vi "Image Difference Main Page.vi"(8 "error in (no error)":errorcluster, 11 "Node Ptr":T3 format="%.0x") -> (0 "error out":errorcluster)   [LabVIEW 2012, in "Image Difference Custom Device.lvlib"]
uses:
  Image Difference Custom Device.lvlib
  <vilib>/NI Veristand/Custom Device API/Custom Device Item Ref.ctl
  <vilib>/userdefined/High Color/IMAQdx.ctl
  TypeDefs/Image Difference State Variables.ctl
  <vilib>/vision/Image Controls.llb/IMAQ Image.ctl
  <vilib>/NI/AMC/Read Next Message.vi
  <vilib>/NI/AMC/Send Local Message.vi
  <vilib>/NI/AMC/Send Local Messages.vi
  <vilib>/NI/AMC/Read Termination Message.vi
  <vilib>/NI/AMC/Create Single Message.vi
  <vilib>/NI/AMC/Update Message Routing Info.vi
  <vilib>/NI/AMC/Create Multiple Messages.vi
  <vilib>/NI/AMC/Create Message Queue.vi
  <vilib>/NI/AMC/Globals.vi
  <vilib>/NI/AMC/Send Message.vi
  Image Difference Global.vi
  <vilib>/NI Veristand/Custom Device API/Set Item Property (String).vi
  <vilib>/NI Veristand/Custom Device API/Set Item Property (Variant).vi
  <vilib>/NI Veristand/Custom Device API/Get Item Property (Variant).vi
  <vilib>/NI Veristand/Custom Device API/Get Item Property (String).vi
  <vilib>/NI/AMC/Destroy Message Queue.vi
  <vilib>/NI Veristand/Custom Device API/Custom Device API.lvlib
  <vilib>/vision/driver/NI_Vision_Acquisition_Software.lvlib
panel:
  in  "Snap Camera":bool
  in  "Camera Session":T1 caption="Session Out"
  out "Camera Image":T2(plugin-control)
  in  "Reset ROI":bool
  in  "Commit ROI":bool
  in  "LoadImage":bool
  in  "Header":cluster{"Section Name":string}={"Section Name"="Custom Device Item Settings"}
  in  "Name":string
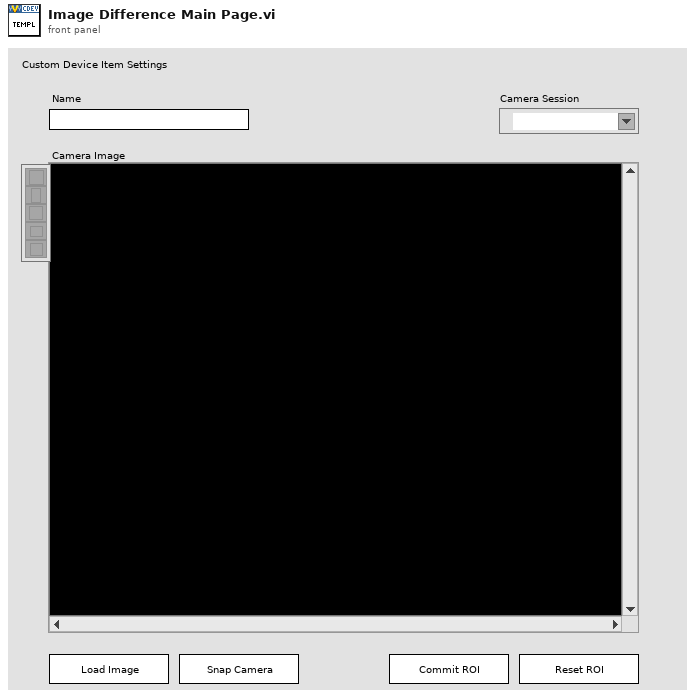
[diagram p1: front panel]
types:
  T1 = typedef "IMAQdx.ctl" = refnum<k21>
  T2 = typedef "IMAQ Image.ctl" = refnum<image>
  T3 = typedef "Custom Device API.lvlib/Custom Device Item Ref.ctl" = u64
  T4 = typedef "Image Difference Custom Device.lvlib/Image Difference State Variables.ctl" = cluster{"NIVS Event":refnum<event-registration>, "Image ROI":cluster{"Global Rectangle":i32[], "Contours":cluster{"Contour Type":u32, "ROI Type":u32, "Points":i32[]}[]}, "Camera Image":T2, "Mouse Depressed?":bool, "Camera Path":string}
  T5 = typedef "AMC.lvlib/Message Queue.ctl" = refnum<queue>
  T6 = typedef "Custom Device API.lvlib/Custom Device Commands.ctl" = enum16{"Default", "Item renamed", "Shutdown", "Dynamic button pressed"}
  T7 = typedef "Custom Device API.lvlib/Custom Device Item Info.ctl" = cluster{"Name":string, "Is Channel":bool, "GUID":string, "Is Waveform":bool}
  T8 = cluster{"Global Rectangle":i32[], "Contours":cluster{"Contour Type":u32, "ROI Type":u32, "Points":i32[]}[]}
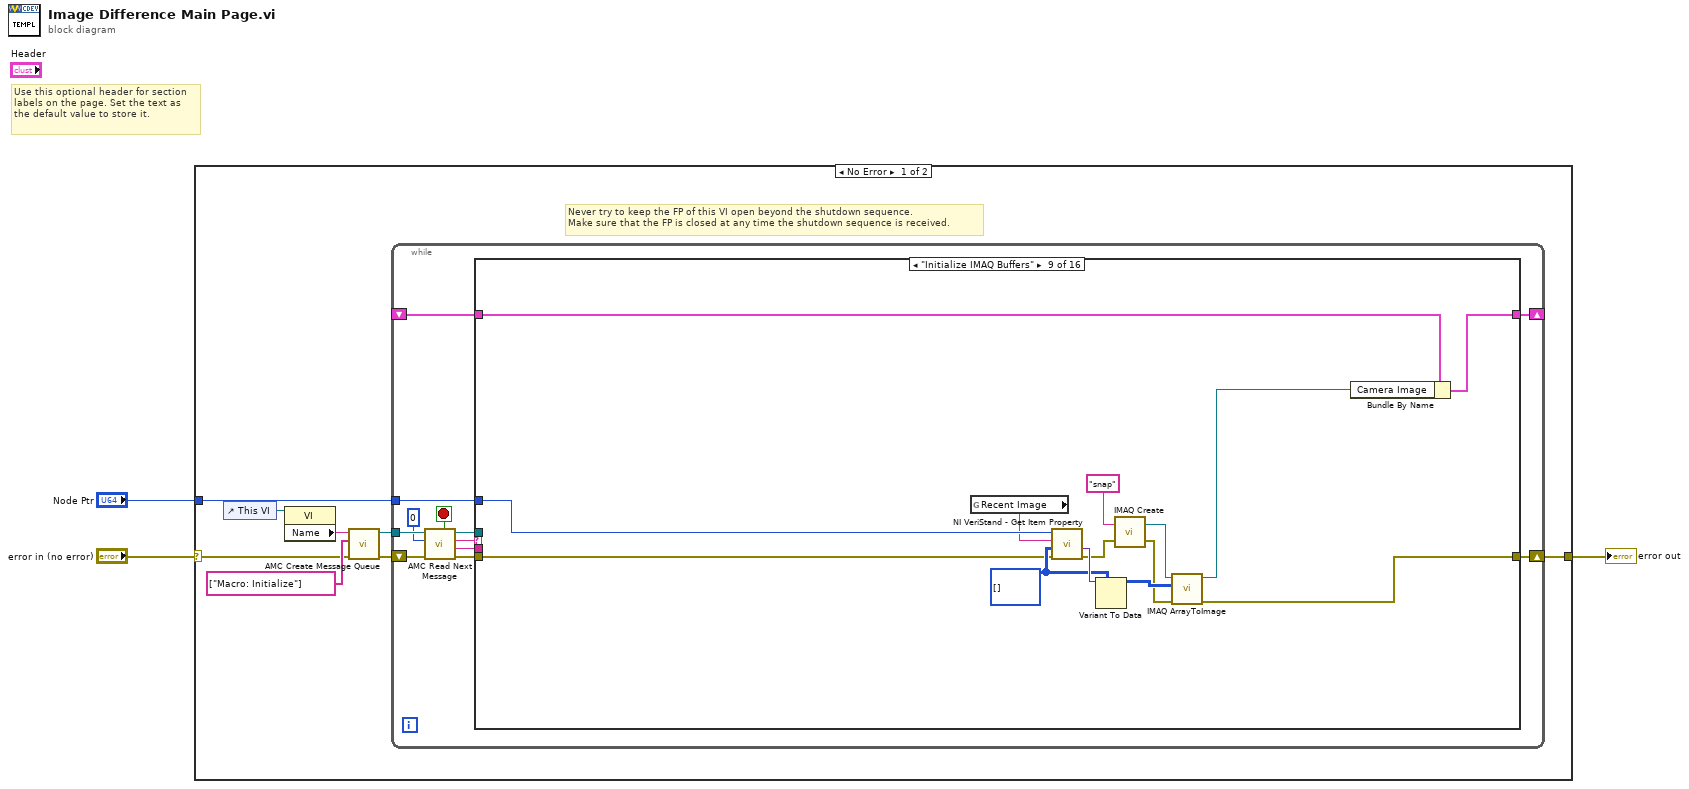
[diagram p0: block diagram]
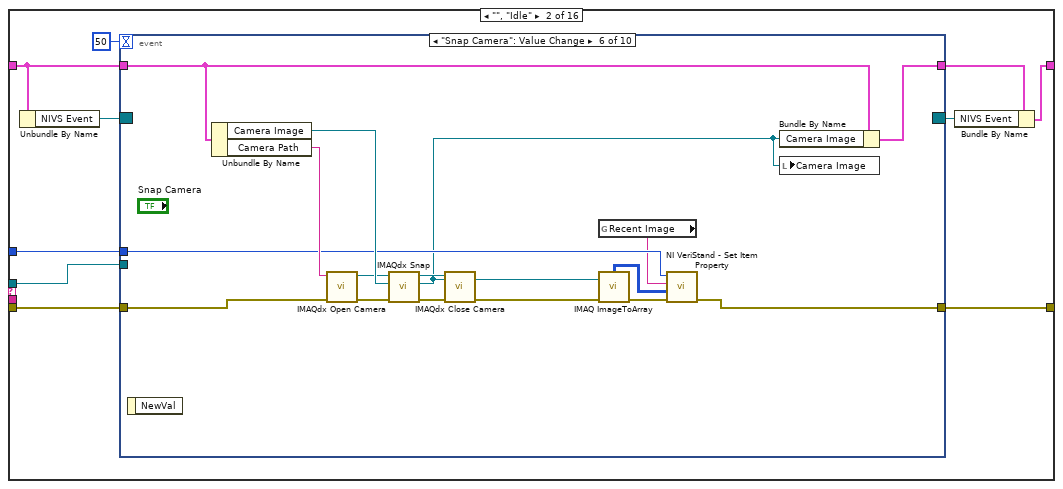
[diagram p3: hidden frame]
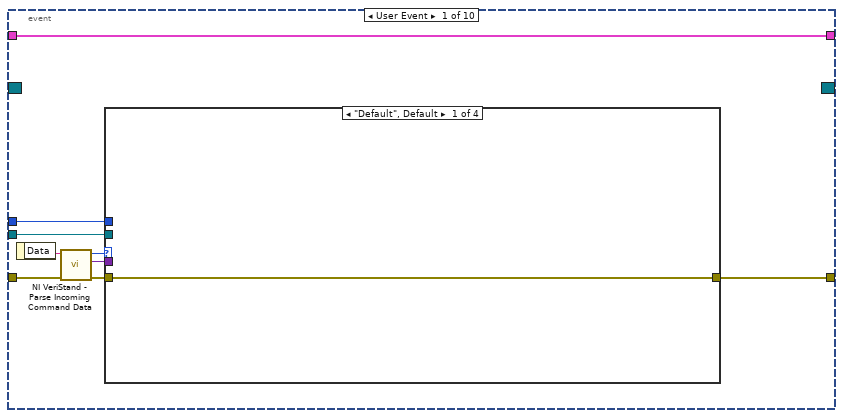
[diagram p4: hidden frame]
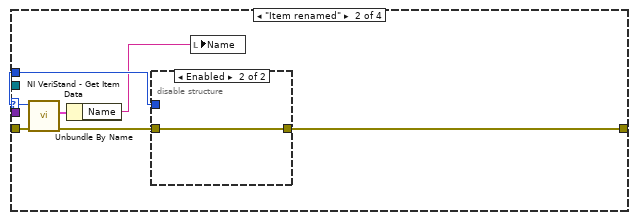
[diagram p5: hidden frame]
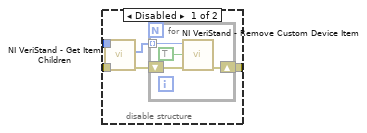
[diagram p6: hidden frame]
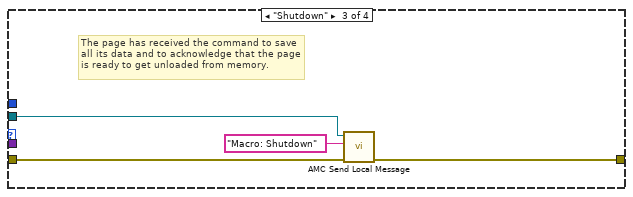
[diagram p7: hidden frame]
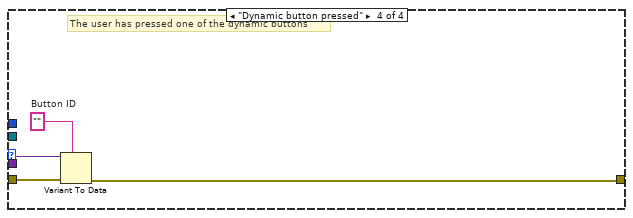
[diagram p8: hidden frame]
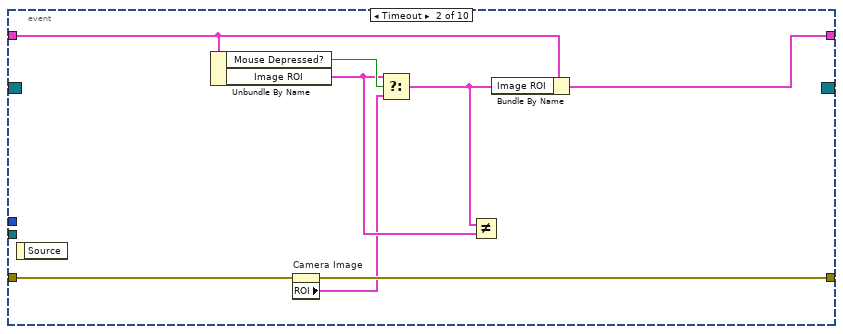
[diagram p9: hidden frame]
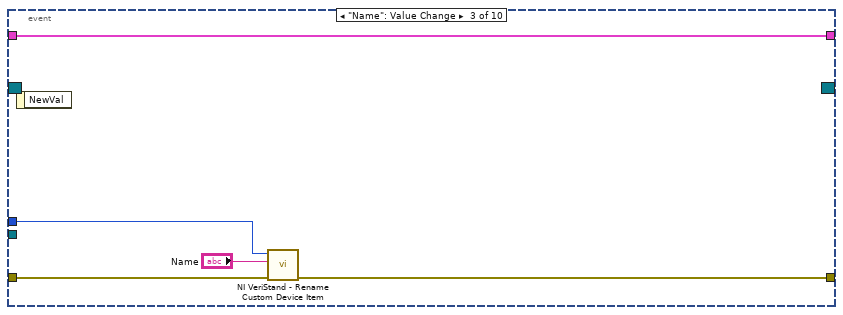
[diagram p10: hidden frame]
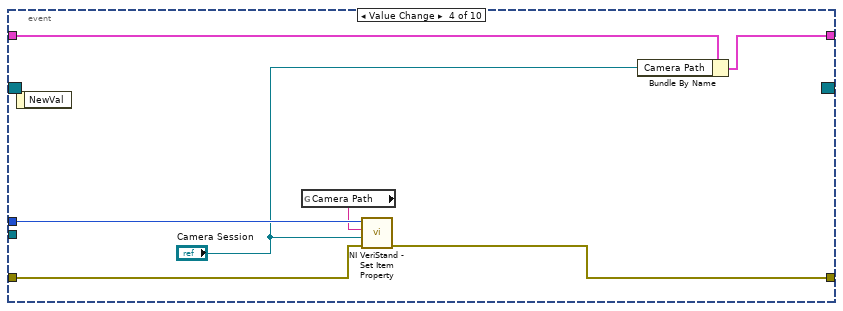
[diagram p11: hidden frame]
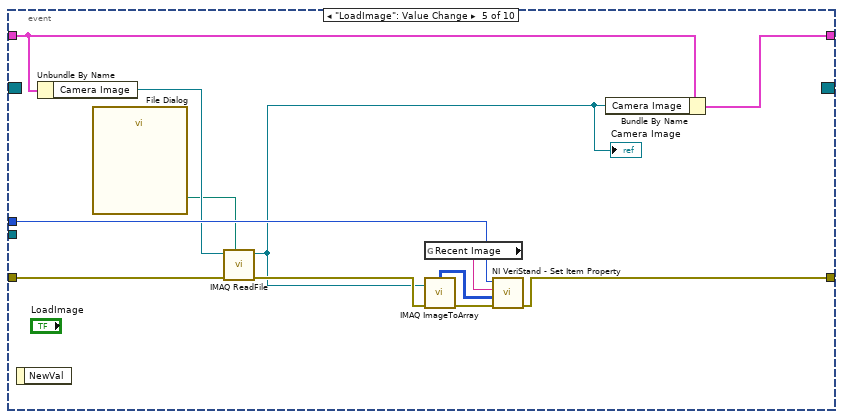
[diagram p12: hidden frame]
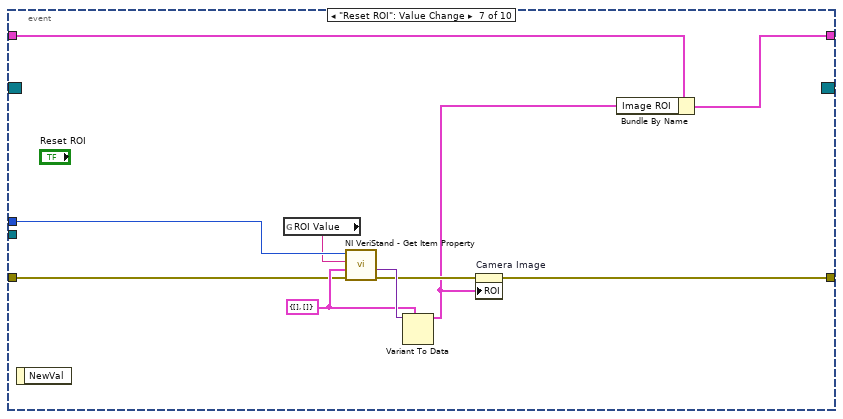
[diagram p13: hidden frame]
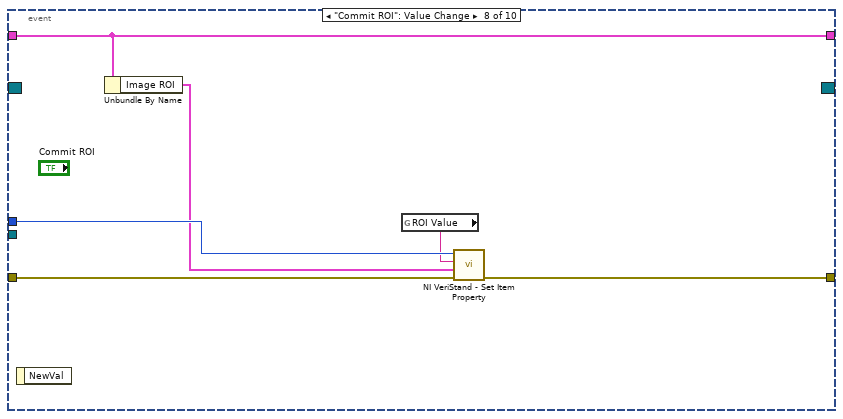
[diagram p14: hidden frame]
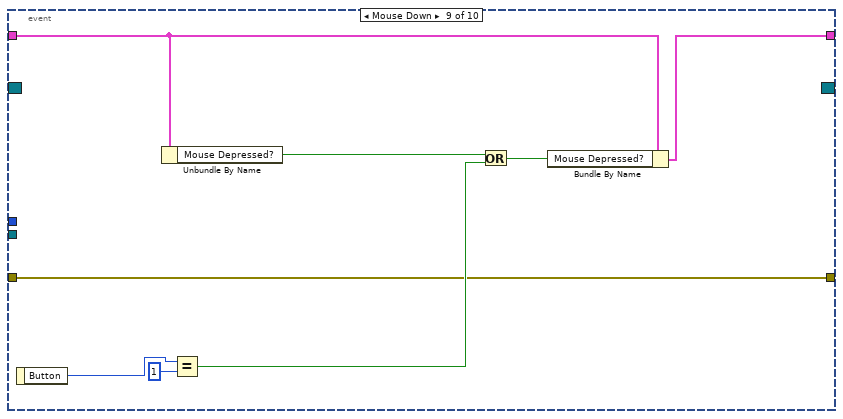
[diagram p15: hidden frame]
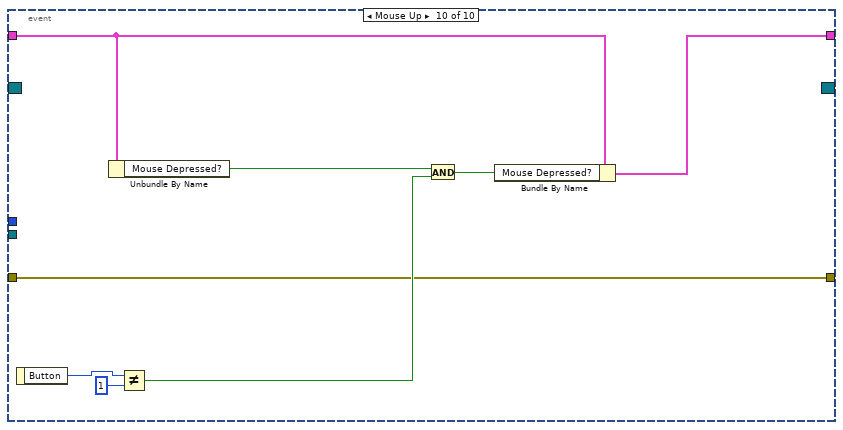
[diagram p16: hidden frame]
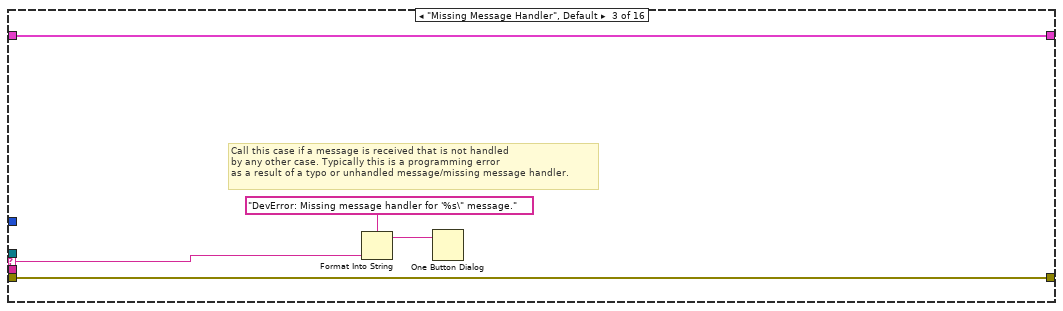
[diagram p17: hidden frame]
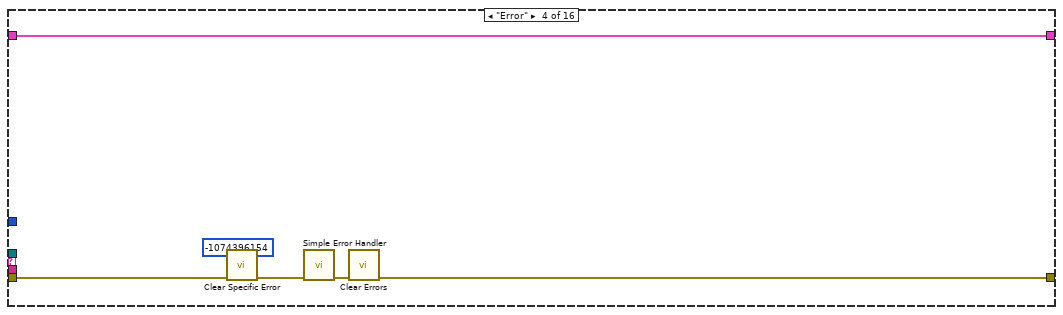
[diagram p18: hidden frame]
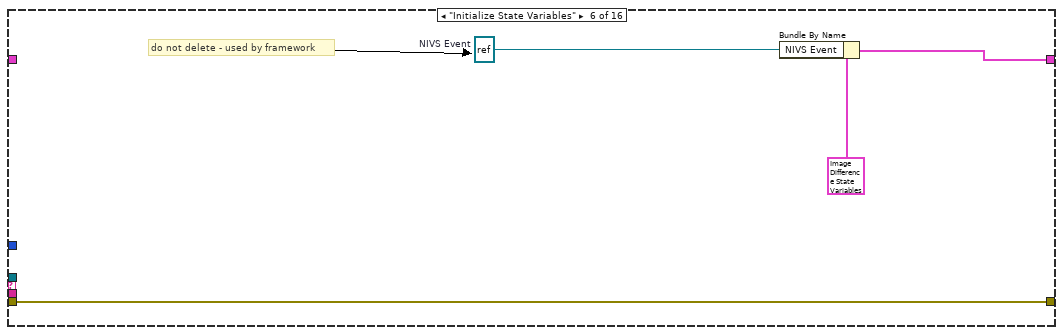
[diagram p20: hidden frame]
diagram:
  # "Use this optional header for section labels on the page. Set the text as the default value to store it."
  n1 = case shown="No Error" "error in (no error)" {
    selector: "error in (no error)" -> [w8 w246]
    tunnel: [w10 w244] -> w1
    tunnel: "Node Ptr" -> [w11 _]
    frame No Error {
      # "Never try to keep the FP of this VI open beyond the shutdown sequence.\nMake sure that the FP is closed at any time the shutdown sequence is received."
      n2 = control-ref of="This VI"() -> (w5:refnum<vi>)
      n3 = property class="VI"(reference=w5) -> ("Name"=w4:string)  [unwired: 1 in, 2 out]
      n4 = call <vilib>:"AMC Create Message Queue.vi"("error in (no error)"=w8, "Initial Message Names"=string[] ["Macro: Initialize"], "Message Queue Name"=w4) -> ("error out"=w7:errorcluster, "Message Queue out"=w6:T5)  [unwired: 1 in, 6 out]
      n5 = while {
        tunnel: w11 -> [w23]
        shift-right: [w20] -> w10
        shift-left: w7 -> [w19]
        shift-right: [w21] -> _
        shift-left: _ -> [w22]
        tunnel: w6 -> [w17]
        stop <- w14 stop-if-true
        n6 = call <vilib>:"AMC Read Next Message.vi"("error in (no error)"=w19, "timeout (1ms)"=0, "Message Queue in"=w17) -> ("error out"=w18:errorcluster, "Message Value"=w13:string, "Message Name"=w12:string, "Message Queue out"=w16:T5, "Exit Process"=w14:bool)  [unwired: 1 in, 3 out]
        n7 = case shown="\"Initialize IMAQ Buffers\"" w12 {
          selector: w12 -> [_ _ w152 _ _ _ _ _ _ _ _ _ _ _ _ _]
          tunnel: w18 -> [w24 w32 w150 w156 w161 w166 w171 w177 w189 w205 w218 w224 w230 w235 w240 w242]
          tunnel: w23 -> [_ w30 _ _ _ _ _ w179 w190 w202 _ _ _ _ _ _]
          tunnel: w22 -> [w25 w28 w151 w158 w162 _ w169 w186 w192 w201 w221 w225 w231 w236 w241 w243]
          tunnel: [w25 w35 w151 w158 w162 w163 w167 w185 w199 w201 w221 w225 w231 w236 w241 w243] -> w21
          tunnel: [w24 w29 w150 w159 w161 w166 w170 w181 w188 w203 w219 w226 w230 w232 w239 w242] -> w20
          tunnel: w16 -> [_ w31 _ _ _ _ _ _ _ _ _ w222 _ w234 w238 _]
          tunnel: w13 -> [_ _ _ _ _ _ _ _ _ _ _ _ _ _ _ _]
          frame "---------- Framework Operations ----------" {
            # "Dummy case to add a seperator in the Case Structure menu"
          }
          frame "", "Idle" {
            n8 = Unbundle By Name(w28) -> ("NIVS Event"=w34:refnum<event-registration>)
            n9 = event shown="[5] \"Snap Camera\": Value Change" {
              selector: w34 -> [_ _ _ _ _ _ _ _ _ _]
              dyn-events: [_ _ _ _ _ _ _ _ _ _] -> w33
              timeout: 50 -> [_ _ _ _ _ _ _ _ _ _]
              tunnel: w32 -> [w44 w75 w82 w88 w95 w109 w123 w131 w134 w142]
              tunnel: [w40 w74 w81 w86 w96 w106 w118 w133 w134 w142] -> w29
              tunnel: w30 -> [w39 _ w80 w89 w97 w105 w122 w132 _ _]
              tunnel: w31 -> [w37 _ _ _ _ _ _ _ _ _]
              tunnel: w28 -> [w36 w77 w79 w85 w99 w107 w127 w130 w135 w144]
              tunnel: [w36 w76 w79 w84 w98 w108 w126 w130 w136 w143] -> w27
              event User Event {
                n10 = event-data() -> ("Data"=w43:string)  [unwired: 1 out]
                n11 = call <vilib>:"NI VeriStand - Parse Incoming Command Data.vi"("error in (no error)"=w44, "Incoming data"=w43) -> ("error out"=w42:errorcluster, "Outgoing data"=w38:variant, "Action"=w41:T6)  [unwired: 7 out]
                n12 = case shown="\"Default\", Default" w41 {
                  tunnel: w42 -> [w45 w51 w64 w69]
                  tunnel: [w45 w46 w63 w66] -> w40
                  tunnel: w39 -> [_ w48 _ _]
                  tunnel: w38 -> [_ _ _ w68]
                  tunnel: w37 -> [_ _ w62 _]
                  frame "Default", Default {
                  }
                  frame "Item renamed" {
                    n13 = call <vilib>:"NI VeriStand - Get Item Data.vi"("error in (no error)"=w51, "Item Ref in"=w48) -> ("error out"=w49:errorcluster, "Item Info"=w50:T7)  [unwired: 8 out]
                    n14 = Unbundle By Name(w50) -> ("Name"=w47:string)
                    n15 = disable-structure shown="Enabled" {
                      disable-tunnel: w49 -> [w56 w61]
                      disable-tunnel: w48 -> [w54 _]
                      disable-tunnel: [w52 w61] -> w46
                      frame Disabled {
                        n16 = call <vilib>:"NI VeriStand - Get Item Children.vi"("error in (no error)"=w56, "Item Ref in"=w54) -> ("error out"=w55:errorcluster, "Child Refs"=w53:T3[])  [unwired: 6 in, 2 out]
                        n17 = for {
                          shift-right: [w58] -> w52
                          shift-left: w55 -> [w60]
                          tunnel: w53 -> [w57] mode=indexing
                          n18 = call <vilib>:"NI VeriStand - Remove Custom Device Item.vi"("error in (no error)"=w60, "Force Delete (F)"=TRUE, "Item Ref in"=w57) -> ("error out"=w58:errorcluster)  [unwired: 7 in, 1 out]
                        }
                      }
                      frame Enabled {
                      }
                    }
                    n19 = local write "Name"(w47) -> ()
                  }
                  frame "Shutdown" {
                    # "The page has received the command to save all its data and to acknowledge that the page is ready to get unloaded from memory."
                    n20 = call <vilib>:"AMC Send Local Message.vi"("error in (no error)"=w64, "Message Name"="Macro: Shutdown", "Message Queue in"=w62) -> ("error out"=w63:errorcluster)  [unwired: 7 in, 1 out]
                  }
                  frame "Dynamic button pressed" {
                    w67 = ""  # Button ID
                    # "The user has pressed one of the dynamic buttons"
                    n21 = Variant To Data(error in=w69, type=w67, Variant=w68) -> (error out=w66:errorcluster)  [unwired: 1 out]
                  }
                }
              }
              event Timeout {
                n22 = event-data() -> ()  [unwired: 2 out]
                n23 = Unbundle By Name(w77) -> ("Mouse Depressed?"=w73:bool, "Image ROI"=w72:T8)
                n24 = property on="Camera Image" class="ImageControl"(error in=w75) -> (error out=w74:errorcluster, "ROI"=w70:T8)  [unwired: 1 in, 1 out]
                n25 = Select(t=w72, s=w73, f=w70) -> (s? t:f=w71:T8)
                n26 = Not Equal?(x=w71, y=w72) -> ()  [unwired: 1 out]
                n27 = Bundle By Name(cluster=w77, "Image ROI"=w71) -> (w76:T4)
              }
              event "Name": Value Change {
                n28 = event-data() -> ()  [unwired: 2 out]
                n29 = call <vilib>:"NI VeriStand - Rename Custom Device Item.vi"("error in (no error)"=w82, "New Name"="Name", "Item Ref in"=w80) -> ("error out"=w81:errorcluster)  [unwired: 1 in, 7 out]
              }
              event Value Change {
                n30 = event-data() -> ()  [unwired: 2 out]
                n31 = global read "Image Difference Global.vi" "Camera Path"() -> (w87:string)
                n32 = call-poly <vilib>:"NI VeriStand - Set Item Property.vi"("error in (no error)"=w88, "Value"="Camera Session", "Property Name"=w87, "Item Ref in"=w89) -> ("error out"=w86:errorcluster)  [unwired: 5 in, 2 out]
                n33 = Bundle By Name(cluster=w85, "Camera Path"="Camera Session") -> (w84:T4)
              }
              event "LoadImage": Value Change {
                n34 = event-data() -> ()  [unwired: 2 out]
                n35 = Unbundle By Name(w99) -> ("Camera Image"=w92:T2)
                n36 = call "File Dialog"() -> ("selected path"=w91:path)  [unwired: 12 in, 3 out]
                n37 = call "IMAQ ReadFile"("File Path"=w91, "error in (no error)"=w95, "Image"=w92) -> ("error out"=w94:errorcluster, "Image Out"=w93:T2)  [unwired: 4 in, 3 out]
                "Camera Image" <- w93
                n38 = global read "Image Difference Global.vi" "Recent Image"() -> (w90:string)
                n39 = call "IMAQ ImageToArray"("error in (no error)"=w94, "Image"=w93) -> ("error out"=w100:errorcluster, "Image Pixels (U8)"=w101:u8[][])  [unwired: 2 in, 3 out]
                n40 = call-poly <vilib>:"NI VeriStand - Set Item Property.vi"("error in (no error)"=w100, "Value"=w101, "Property Name"=w90, "Item Ref in"=w97) -> ("error out"=w96:errorcluster)  [unwired: 5 in, 2 out]
                n41 = Bundle By Name(cluster=w99, "Camera Image"=w93) -> (w98:T4)
              }
              event "Snap Camera": Value Change {
                n42 = event-data() -> ()  [unwired: 2 out]
                n43 = Unbundle By Name(w107) -> ("Camera Image"=w117:T2, "Camera Path"=w116:string)
                n44 = call <vilib>:"IMAQdx Open Camera.vi"("error in"=w109, "Session In"=w116) -> ("error out"=w110:errorcluster, "Session Out"=w111:T1)  [unwired: 8 in]
                n45 = call <vilib>:"IMAQdx Snap.vi"("error in"=w110, "Image In"=w117, "Session In"=w111) -> ("error out"=w112:errorcluster, "Image Out"=w103:T2, "Session Out"=w113:T1)  [unwired: 6 in]
                n46 = call <vilib>:"IMAQdx Close Camera.vi"("error in"=w112, "Session In"=w113) -> ("error out"=w104:errorcluster)  [unwired: 9 in]
                n47 = global read "Image Difference Global.vi" "Recent Image"() -> (w102:string)
                n48 = call "IMAQ ImageToArray"("error in (no error)"=w104, "Image"=w103) -> ("error out"=w115:errorcluster, "Image Pixels (U8)"=w114:u8[][])  [unwired: 2 in, 3 out]
                n49 = call-poly <vilib>:"NI VeriStand - Set Item Property.vi"("error in (no error)"=w115, "Value"=w114, "Property Name"=w102, "Item Ref in"=w105) -> ("error out"=w106:errorcluster)  [unwired: 5 in, 2 out]
                n50 = Bundle By Name(cluster=w107, "Camera Image"=w103) -> (w108:T4)
                n51 = local write "Camera Image"(w103) -> ()
              }
              event "Reset ROI": Value Change {
                w124 = T8 {"Global Rectangle"=[], "Contours"=[]} ("ROI")
                n52 = event-data() -> ()  [unwired: 2 out]
                n53 = global read "Image Difference Global.vi" "ROI Value"() -> (w119:string)
                n54 = call-poly <vilib>:"NI VeriStand - Get Item Property.vi"("error in (no error)"=w123, "Default Value"=w124, "Property Name"=w119, "Item Ref in"=w122) -> ("error out"=w121:errorcluster, "Value"=w125:variant)  [unwired: 4 in, 2 out]
                n55 = Variant To Data(type=w124, Variant=w125) -> (data=w120:T8)  [unwired: 1 in, 1 out]
                n56 = property on="Camera Image" class="ImageControl"(error in=w121, "ROI"=w120) -> (error out=w118:errorcluster)  [unwired: 1 in, 1 out]
                n57 = Bundle By Name(cluster=w127, "Image ROI"=w120) -> (w126:T4)
              }
              event "Commit ROI": Value Change {
                n58 = event-data() -> ()  [unwired: 2 out]
                n59 = Unbundle By Name(w130) -> ("Image ROI"=w129:T8)
                n60 = global read "Image Difference Global.vi" "ROI Value"() -> (w128:string)
                n61 = call-poly <vilib>:"NI VeriStand - Set Item Property.vi"("error in (no error)"=w131, "Value"=w129, "Property Name"=w128, "Item Ref in"=w132) -> ("error out"=w133:errorcluster)  [unwired: 5 in, 2 out]
              }
              event Mouse Down {
                n62 = event-data() -> ("Button"=w137:u16)  [unwired: 1 out]
                n63 = Unbundle By Name(w135) -> ("Mouse Depressed?"=w141:bool)
                n64 = Equal?(x=w137, y=u16 1) -> (x = y?=w139:bool)
                n65 = Or(x=w141, y=w139) -> (x .or. y?=w140:bool)
                n66 = Bundle By Name(cluster=w135, "Mouse Depressed?"=w140) -> (w136:T4)
              }
              event Mouse Up {
                n67 = event-data() -> ("Button"=w145:u16)  [unwired: 1 out]
                n68 = Unbundle By Name(w144) -> ("Mouse Depressed?"=w149:bool)
                n69 = Not Equal?(x=w145, y=u16 1) -> (x != y?=w147:bool)
                n70 = And(x=w149, y=w147) -> (x .and. y?=w148:bool)
                n71 = Bundle By Name(cluster=w144, "Mouse Depressed?"=w148) -> (w143:T4)
              }
            }
            n72 = Bundle By Name(cluster=w27, "NIVS Event"=w33) -> (w35:T4)
          }
          frame "Missing Message Handler", Default {
            # "Call this case if a message is received that is not handled \nby any other case. Typically this is a programming error\nas a result of a typo or unhandled message/missing message handler."
            n73 = Format Into String(format string="DevError: Missing message handler for '%s\" message." ("message"), w152) -> (resulting string=w154:string)  [unwired: 2 in, 1 out]
            n74 = One Button Dialog(message=w154) -> ()  [unwired: 2 out]
          }
          frame "Error" {
            n75 = call "Clear Specific Error.vi"("Error to Clear"=-1074396154, "Error In"=w156) -> ("Error Out"=w155:errorcluster)  [unwired: 6 in, 1 out]
            n76 = call <vilib>:"Simple Error Handler.vi"("error in (no error)"=w155) -> ("error out"=w160:errorcluster)  [unwired: 1 in, 7 out]
            n77 = call <vilib>:"Clear Errors.vi"("error in (no error)"=w160) -> ("error out"=w159:errorcluster)  [unwired: 6 out]
          }
          frame "---------- Init/Shutdown Operations ----------" {
            # "Dummy case to add a seperator in the Case Structure menu"
          }
          frame "Initialize State Variables" {
            w164 = refnum<event-registration> refnum  # NIVS Event
            # "do not delete - used by framework"
            n78 = Bundle By Name(cluster=T4 {"NIVS Event"=refnum, "Image ROI"={"Global Rectangle"=[], "Contours"=[]}, "Camera Image"=refnum, "Mouse Depressed?"=FALSE, "Camera Path"=""} ("State Variables"), "NIVS Event"=w164) -> (w163:T4)
          }
          frame "Initialize Core Data" {
            # "Do Not Delete. This initializes the event registration for the event structure."
            n79 = call <vilib>:"NI VeriStand - Get Event Refnum.vi"("error in (no error)"=w171) -> ("error out"=w172:errorcluster, "Event Ref"=w173:refnum<user-event>)  [unwired: 9 out]
            n80 = register-events(error in=w172, w173) -> (reference out=w168:refnum<event-registration>, error out=w170:errorcluster)  [unwired: 1 in]
            n81 = Bundle By Name(cluster=w169, "NIVS Event"=w168) -> (w167:T4)
          }
          frame "Initialize Item Properties" {
            w184 = T8 {"Global Rectangle"=[], "Contours"=[]} ("ROI")
            n82 = global read "Image Difference Global.vi" "Camera Path"() -> (w175:string)
            n83 = call-poly <vilib>:"NI VeriStand - Get Item Property.vi"("error in (no error)"=w177, "Property Name"=w175, "Item Ref in"=w179) -> ("error out"=w176:errorcluster, "Value"=w174:string, "Item Ref out"=w178:T3)  [unwired: 5 in, 1 out]
            n84 = global read "Image Difference Global.vi" "ROI Value"() -> (w180:string)
            n85 = call-poly <vilib>:"NI VeriStand - Get Item Property.vi"("error in (no error)"=w176, "Default Value"=w184, "Property Name"=w180, "Item Ref in"=w178) -> ("error out"=w181:errorcluster, "Value"=w183:variant)  [unwired: 4 in, 2 out]
            n86 = Variant To Data(type=w184, Variant=w183) -> (data=w182:T8)  [unwired: 1 in, 1 out]
            n87 = Bundle By Name(cluster=w186, "Camera Path"=w174, "Image ROI"=w182) -> (w185:T4)
          }
          frame "Initialize IMAQ Buffers" {
            w197 = u8[][] []
            n88 = global read "Image Difference Global.vi" "Recent Image"() -> (w187:string)
            n89 = call-poly <vilib>:"NI VeriStand - Get Item Property.vi"("error in (no error)"=w189, "Default Value"=w197, "Property Name"=w187, "Item Ref in"=w190) -> ("error out"=w195:errorcluster, "Value"=w198:variant)  [unwired: 4 in, 2 out]
            n90 = Variant To Data(type=w197, Variant=w198) -> (data=w196:u8[][])  [unwired: 1 in, 1 out]
            n91 = call "IMAQ Create"("Image Name"="snap", "error in (no error)"=w195) -> ("New Image"=w193:T2, "error out"=w194:errorcluster)  [unwired: 3 in]
            n92 = call "IMAQ ArrayToImage"("error in (no error)"=w194, "Image Pixels (U8)"=w196, "Image"=w193) -> ("error out"=w188:errorcluster, "Image Out"=w191:T2)  [unwired: 7 in]
            n93 = Bundle By Name(cluster=w192, "Camera Image"=w191) -> (w199:T4)
          }
          frame "Initialize User Interface" {
            n94 = flat-sequence "Initialize UI Frame" {
              tunnel: w205 -> [w214]
              tunnel: [w210] -> w204
              tunnel: w202 -> [w215]
              tunnel: w201 -> [w213]
              frame #0 {
                w206 = u32 3 items=["Zoom Tool"=8, "Selection Tool"=0, "Pan Tool"=9, "Point Tool"=1, "Line Tool"=2, "Rectangle Tool"=3, "Rotated Rectangle Tool"=12, "Polyline Tool"=10, "Polygon Tool"=5, "Freehand Tool"=11, "Closed Freehand Tool"=6, "Ellipse Tool"=4, "Annulus Tool"=7] ("Current ROI Tool")
                # "NI recommends to initialize the page up front\nand to release the FP cursor afterwards.\nTo release the FP cursor is mandatory!"
                # "Initialize all UI Elements Here"
                n95 = call <vilib>:"NI VeriStand - Get Item Data.vi"("error in (no error)"=w214, "Item Ref in"=w215) -> ("error out"=w211:errorcluster, "Item Info"=w216:T7)  [unwired: 8 out]
                n96 = Unbundle By Name(w216) -> ("Name"=w217:string)
                n97 = Unbundle By Name(w213) -> ("Camera Path"=w208:string, "Camera Image"=w212:T2, "Image ROI"=w209:T8)
                n98 = local write "Name"(w217) -> ()
                n99 = local write "Camera Session"(w208) -> ()
                n100 = local write "Camera Image"(w212) -> ()
                n101 = property on="Camera Image" class="ImageControl"(error in=w211, "ROI"=w209) -> (error out=w210:errorcluster)  [unwired: 1 in, 1 out]
                n102 = property on="Camera Image" class="ImageControl"("Zoom to Fit Mode"=TRUE, "Current ROI Tool"=w206) -> ()  [unwired: 2 in, 2 out]
              }
            }
            n103 = call <vilib>:"NI VeriStand - Unset Busy Cursor.vi"("error in (no error)"=w204) -> ("error out"=w203:errorcluster)  [unwired: 10 out]
          }
          frame "Data Cleanup" {
            # "Cleanup all data and references here."
            n104 = Unbundle By Name(w221) -> ("Camera Image"=w220:T2)
            n105 = call "IMAQ Dispose"("Image"=w220, "error in (no error)"=w218) -> ("error out"=w219:errorcluster)  [unwired: 4 in]
          }
          frame "Exit" {
            n106 = call <vilib>:"AMC Destroy Message Queue.vi"("error in (no error)"=w224, "Message Queue in"=w222) -> ("error out"=w223:errorcluster)  [unwired: 9 out]
            n107 = Unbundle By Name(w225) -> ("NIVS Event"=w229:refnum<event-registration>)
            n108 = Unregister For Events(event registration refnum=w229, error in=w223) -> (error out=w228:errorcluster)
            n109 = invoke class="VI" method="FP.Close"(error in=w228) -> (error out=w227:errorcluster)  [unwired: 2 in, 2 out]
            n110 = call <vilib>:"NI VeriStand - Signal When Ready for Shutdown.vi"("error in (no error)"=w227) -> ("error out"=w226:errorcluster)  [unwired: 10 out]
          }
          frame "---------- Macro Operations ----------" {
            # "Dummy case to add a seperator in the Case Structure menu"
          }
          frame "Macro: Initialize" {
            # "Initialization Macro. This is called when VI starts and calls all Init cases."
            n111 = call <vilib>:"AMC Send Local Messages.vi"("error in (no error)"=w235, "Message Names"=string[] ["Initialize State Variables", "Initialize Core Data", "Initialize Item Properties", "Initialize IMAQ Buffers", "Initialize User Interface"], "Message Queue in"=w234) -> ("error out"=w232:errorcluster)  [unwired: 7 in, 1 out]
          }
          frame "Macro: Shutdown" {
            # "Shutdown Macro. This is called when VI shuts down and calls all shutdown cases"
            n112 = call <vilib>:"AMC Send Local Messages.vi"("error in (no error)"=w240, "Message Names"=string[] ["Data Cleanup", "Exit"], "Message Queue in"=w238) -> ("error out"=w239:errorcluster)  [unwired: 7 in, 1 out]
          }
          frame "---------- Application Operations ----------" {
            # "Dummy case to add a seperator in the Case Structure menu"
          }
        }
      }
    }
    frame Error {
      n113 = call <vilib>:"Simple Error Handler.vi"("error in (no error)"=w246) -> ("error out"=w245:errorcluster)  [unwired: 1 in, 7 out]
      n114 = call <vilib>:"Clear Errors.vi"("error in (no error)"=w245) -> ("error out"=w244:errorcluster)  [unwired: 6 out]
    }
  }
  "error out" <- w1
